vi "R_W Command - Asynchronous.vi"(8 "error in":errorcluster, 9 "Query?":bool=TRUE, 10 "Command":string="SYST:COMM:HAND", 11 "SCPI in":refnum<class "SCPI.lvclass">) -> (0 "error out":errorcluster, 2 "read buffer":string, 3 "SCPI out":refnum<class "SCPI.lvclass">)   [LabVIEW 2011, in "SCPI.lvclass"]
doc: "Basic command for R/W on SCPI. This is just essentially a call to the serial asynchronous R/W with the addition of a query option. The query will tack on a ? at the end of the command."
uses:
  SCPI.lvclass
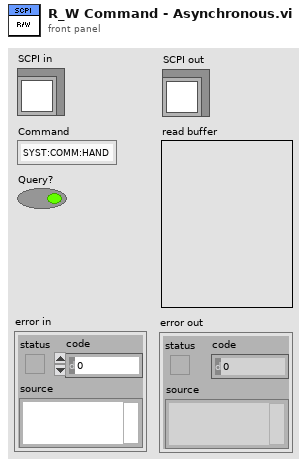
[diagram p1: front panel]
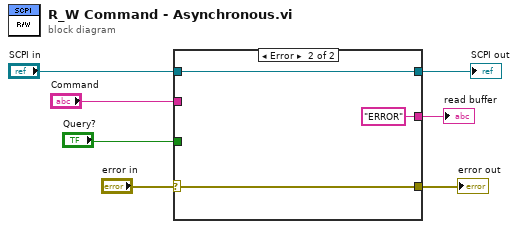
[diagram p0: block diagram]
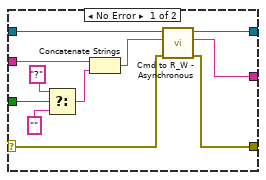
[diagram p2: hidden frame]
diagram:
  n1 = case shown="Error" "error in" {
    selector: "error in" -> [w16 w21]
    tunnel: [w15 w21] -> w1
    tunnel: [w17 w20] -> w3
    tunnel: "SCPI in" -> [w18 w20]
    tunnel: "Query?" -> [w14 _]
    tunnel: "Command" -> [w10 _]
    tunnel: [w8 "ERROR" ("read buffer")] -> w5
    frame No Error {
      n2 = Select(t="?", s=w14, f="") -> (s? t:f=w11:string)
      n3 = Concatenate Strings(w10, w11) -> (w9:string)
      n4 = call-dynamic "Cmd to R_W - Asynchronous.vi"("error in"=w16, "write buffer"=w9, "Serial IO in"=w18) -> ("error out"=w15:errorcluster, "read buffer"=w8:string, "Serial IO out"=w17:refnum<class "SCPI.lvclass">)  [unwired: 6 in]
    }
    frame Error {
    }
  }
  "error out" <- w1
  "SCPI out" <- w3
  "read buffer" <- w5
